vi "send_to_all_processes.vi"(8 "error in (no error)":errorcluster, 9 "Control_process_state_cluster in":T1={"Control_process_state_enum"=enum."Stop", "variant"=variant}, 10 "Process names":string[](array[string]), 11 "Process_communication in":variant) -> (0 "error out":errorcluster, 3 "Process_communication out":variant)   [LabVIEW 2011, in "Fiberscope_library.lvlib"]
uses:
  Fiberscope_library.lvlib
  typedefs/control_process_state_cluster.ctl
  typedefs/control_process_state_enum.ctl
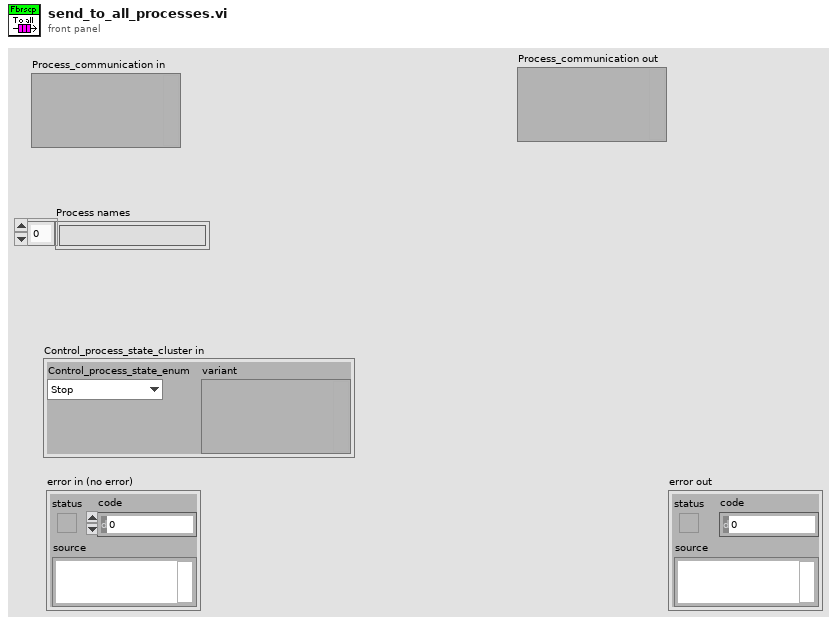
[diagram p1: front panel]
types:
  T1 = typedef "Fiberscope_library.lvlib/control_process_state_cluster.ctl" = cluster{"Control_process_state_enum":T2, "variant":variant}
  T2 = typedef "Fiberscope_library.lvlib/control_process_state_enum.ctl" = enum16{"Init", "Quit", "Start", "Stop", "Change_parameters", "Running", "Finish", "Custom"}
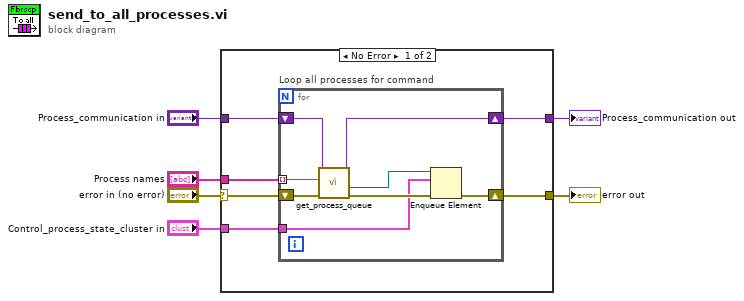
[diagram p0: block diagram]
diagram:
  n1 = case shown="No Error" "error in (no error)" {
    selector: "error in (no error)" -> [w11 w22]
    tunnel: [w7 w22] -> w1
    tunnel: "Control_process_state_cluster in" -> [w10 _]
    tunnel: "Process names" -> [w9 _]
    tunnel: "Process_communication in" -> [w12 w21]
    tunnel: [w8 w21] -> w3
    frame No Error {
      n2 = for "Loop all processes for command" {
        shift-right: [w13] -> w7
        shift-left: w11 -> [w20]
        tunnel: w10 -> [w14]
        tunnel: w9 -> [w18] mode=indexing
        shift-right: [w15] -> w8
        shift-left: w12 -> [w19]
        n3 = call "get_process_queue.vi"("error in (no error)"=w20, "Process name"=w18, "Process_communication in"=w19) -> ("error out"=w17:errorcluster, "Process_control_queue"=w16:refnum<queue>, "Process_communication out"=w15:variant)  [unwired: 6 in]
        n4 = Enqueue Element(queue=w16, element=w14, error in (no error)=w17) -> (error out=w13:errorcluster)  [unwired: 1 in, 2 out]
      }
    }
    frame Error {
    }
  }
  "error out" <- w1
  "Process_communication out" <- w3
